vi "AddConfigureDialog.vi"(8 "Error In":errorcluster) -> (0 "Error Out":errorcluster)   [LabVIEW 2015]
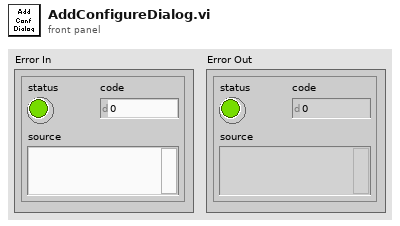
[diagram p1: front panel]
types:
  T1 = enum16{"Invalid Wire Rule", "Required", "Recommended", "Optional", "Dynamic Dispatch"}
  T2 = typedef "LVRectTypeDef.ctl" = cluster{"Left":i16, "Top":i16, "Right":i16, "Bottom":i16}
  T3 = enum16{"Invalid Wire Rule", "Required", "Recommended", "Optional", "Dynamic Dispatch"}[]
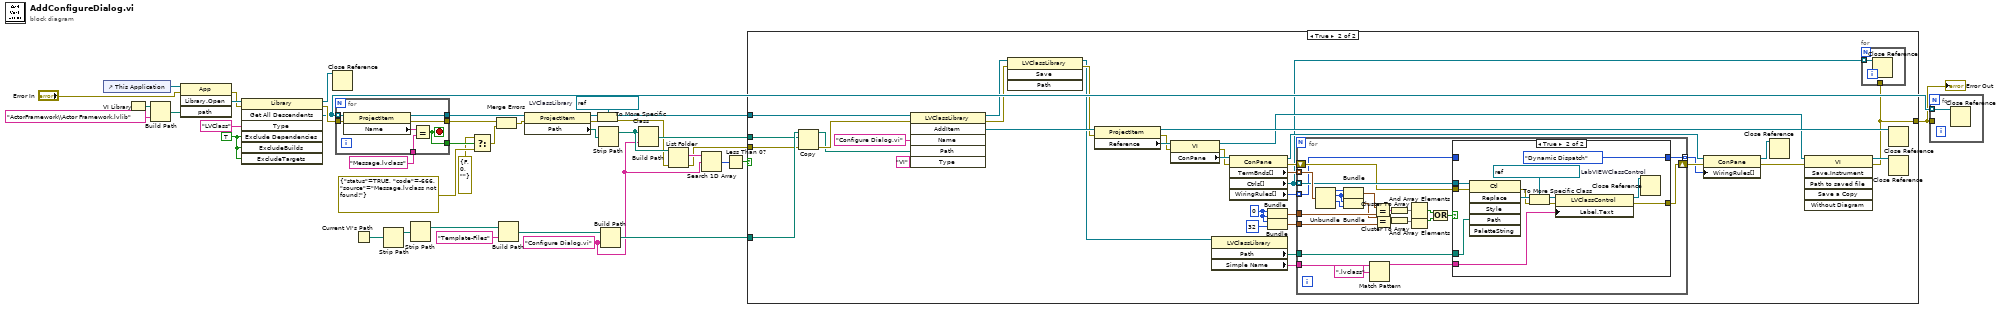
[diagram p0: block diagram]
diagram:
  w17 = refnum<vi> refnum  # LVClassLibrary
  w7 = "Configure Dialog.vi" ("name or relative path")
  w33 = TRUE ("ExcludeDependencies")
  n1 = control-ref of="This Application"() -> (w40:refnum<vi>)
  n2 = VI Library() -> (path=w39:path)
  n3 = Build Path(base path=w39, name or relative path="ActorFramework\\Actor Framework.lvlib") -> (appended path=w37:path)
  n4 = invoke class="App" method="Library.Open"(reference=w40, error in="Error In", "path"=w37) -> (error out=w34:errorcluster, "Open Library"=w35:refnum<vi>)  [unwired: 1 in, 2 out]
  n5 = invoke class="Library" method="Get All Descendents"(reference=w35, error in=w34, "Type"="LVClass", "Exclude Dependencies"=w33, "ExcludeBuilds"=w33, "ExcludeTargets"=w33) -> (reference out=w13:refnum<vi>, error out=w32:errorcluster, "All Descendents"=w12:refnum<vi>[])  [unwired: 1 in, 4 out]
  n6 = Close Reference(reference=w13) -> ()  [unwired: 1 in, 1 out]
  n7 = for {
    tunnel: w12 -> [w47] mode=indexing
    tunnel: "Message.lvclass" ("name") -> [w45]
    tunnel: [w44] -> w21
    tunnel: w32 -> [w43]
    tunnel: [w42] -> w26
    tunnel: [w41] -> w30
    stop <- w41 stop-if-true
    n8 = property class="ProjectItem"(reference=w47, error in=w43) -> (reference out=w44:refnum<vi>, error out=w42:errorcluster, "Name"=w46:string)
    n9 = Equal?(x=w46, y=w45) -> (x = y?=w41:bool)
  }
  n10 = Current VI's Path() -> (path=w25:path)
  n11 = Strip Path(path=w25) -> (stripped path=w24:path)  [unwired: 1 out]
  n12 = Strip Path(path=w24) -> (stripped path=w1:path)  [unwired: 1 out]
  n13 = Select(t=errorcluster {"status"=FALSE, "code"=0, "source"=""} ("error constant"), s=w30, f=errorcluster {"status"=TRUE, "code"=-666, "source"="Message.lvclass not found!"} ("error constant")) -> (s? t:f=w27:errorcluster)
  n14 = Merge Errors(w26, w27) -> (w20:errorcluster)
  n15 = Build Path(base path=w1, name or relative path="Template-Files") -> (appended path=w22:path)
  n16 = property class="ProjectItem"(reference=w21, error in=w20) -> (reference out=w16:refnum<vi>, error out=w14:errorcluster, "Path"=w18:path)
  n17 = To More Specific Class(target class=w17, reference=w16, error in=w14) -> (specific class reference=w15:refnum<vi>, error out=w9:errorcluster)
  n18 = Strip Path(path=w18) -> (stripped path=w10:path)  [unwired: 1 out]
  n19 = Build Path(base path=w22, name or relative path=w7) -> (appended path=w19:path)
  n20 = Build Path(base path=w10, name or relative path=w7) -> (appended path=w11:path)
  n21 = List Folder(path=w10, error in=w9) -> (filenames=w8:string[], error out=w6:errorcluster)  [unwired: 2 in, 2 out]
  n22 = Search 1D Array(1D array=w8, element=w7) -> (index of element=w5:i32)  [unwired: 1 in]
  n23 = Less Than 0?(x=w5) -> (x < 0?=w4:bool)
  n24 = case shown="True" w4 {
    tunnel: w19 -> [_ w78]
    tunnel: w15 -> [_ w76]
    tunnel: [w48 w51] -> w2
    tunnel: w11 -> [_ w50]
    tunnel: w6 -> [w48 w49]
    frame False {
    }
    frame True {
      w64 = i16 0
      n25 = Copy(8:w49, 10:w50, 11:w78) -> (0:w79:errorcluster, 3:w77:path)  [unwired: 2 in, 1 out]
      n26 = invoke class="LVClassLibrary" method="AddItem"(reference=w76, error in=w79, "Name"="Configure Dialog.vi", "Path"=w77, "Type"="VI") -> (reference out=w75:refnum<vi>, error out=w74:errorcluster, "AddItem"=w82:refnum<vi>)  [unwired: 1 in, 3 out]
      n27 = invoke class="LVClassLibrary" method="Save"(reference=w75, error in=w74) -> (reference out=w56:refnum<vi>, error out=w73:errorcluster)  [unwired: 2 in, 2 out]
      n28 = property class="ProjectItem"(reference=w82, error in=w73) -> (reference out=w81:refnum<vi>, error out=w57:errorcluster, "Reference"=w58:refnum<vi>)
      n29 = property class="VI"(reference=w58, error in=w57) -> (reference out=w55:refnum<vi>, error out=w71:errorcluster, "ConPane"=w72:refnum<vi>)
      n30 = property class="LVClassLibrary"(reference=w56) -> ("Path"=w65:path, "Simple Name"=w59:string)  [unwired: 1 in, 2 out]
      n31 = property class="ConPane"(reference=w72, error in=w71) -> (reference out=w61:refnum<vi>, error out=w69:errorcluster, "TermBnds[]"=w70:T2[], "Ctrls[]"=w52:refnum<vi>[], "WiringRules[]"=w63:T3)
      n32 = Bundle(w64, w64) -> (w67:cluster{i16, i16})  [unwired: 1 in]
      n33 = Bundle(w64, i16 32) -> (w66:cluster{i16, i16})  [unwired: 1 in]
      n34 = for {
        tunnel: w70 -> [w108] mode=indexing
        tunnel: w52 -> [w98] mode=indexing
        shift-right: [w92] -> w62
        shift-left: w69 -> [w97]
        tunnel: w67 -> [w105]
        tunnel: w66 -> [w103]
        tunnel: w65 -> [w93]
        tunnel: w63 -> [w89] mode=indexing
        tunnel: [w88] -> w60 mode=indexing
        tunnel: w59 -> [w87]
        n35 = Unbundle(w108) -> ("Left"=w107:i16, "Top"=w90:i16, "Right"=w91:i16)  [unwired: 1 out]
        n36 = Bundle("Left"=w107, "Top"=w90) -> (w106:cluster{"Left":i16, "Top":i16})  [unwired: 1 in]
        n37 = Bundle("Top"=w90, "Right"=w91) -> (w104:cluster{"Top":i16, "Right":i16})  [unwired: 1 in]
        n38 = Match Pattern(string=w87, regular expression=".lvclass") -> (before substring=w86:string)  [unwired: 1 in, 3 out]
        n39 = Equal?(x=w106, y=w105) -> (x = y?=w102:cluster{bool, bool})
        n40 = Equal?(x=w104, y=w103) -> (x = y?=w101:cluster{bool, bool})
        n41 = Cluster To Array(cluster=w102) -> (array=w100:bool[])
        n42 = Cluster To Array(cluster=w101) -> (array=w99:bool[])
        n43 = And Array Elements(Boolean array=w100) -> (logical AND=w96:bool)
        n44 = And Array Elements(Boolean array=w99) -> (logical AND=w95:bool)
        n45 = Or(x=w96, y=w95) -> (x .or. y?=w94:bool)
        n46 = case shown="True" w94 {
          tunnel: w98 -> [_ w122]
          tunnel: w97 -> [w110 w121]
          tunnel: [w110 w113] -> w92
          tunnel: w93 -> [_ w120]
          tunnel: w89 -> [w109 _]
          tunnel: [w109 T1."Dynamic Dispatch" ("Wire Rule")] -> w88
          tunnel: w86 -> [_ w111]
          frame False {
          }
          frame True {
            w118 = refnum<vi> refnum  # LabVIEWClassControl
            n47 = invoke class="Ctl" method="Replace"(reference=w122, error in=w121, "Path"=w120) -> (error out=w114:errorcluster, "Replace"=w117:refnum<vi>)  [unwired: 3 in, 4 out]
            n48 = To More Specific Class(target class=w118, reference=w117, error in=w114) -> (specific class reference=w116:refnum<vi>, error out=w115:errorcluster)
            n49 = property class="LVClassControl"(reference=w116, error in=w115, "Label.Text"=w111) -> (reference out=w112:refnum<vi>, error out=w113:errorcluster)
            n50 = Close Reference(reference=w112) -> ()  [unwired: 1 in, 1 out]
          }
        }
      }
      n51 = property class="ConPane"(reference=w61, error in=w62, "WiringRules[]"=w60) -> (reference out=w53:refnum<vi>, error out=w54:errorcluster)
      n52 = Close Reference(reference=w53) -> ()  [unwired: 1 in, 1 out]
      n53 = invoke class="VI" method="Save.Instrument"(reference=w55, error in=w54) -> (reference out=w80:refnum<vi>, error out=w51:errorcluster)  [unwired: 4 in, 4 out]
      n54 = for {
        tunnel: w52 -> [w123] mode=indexing
        tunnel: w51 -> [_]
        n55 = Close Reference(reference=w123) -> ()  [unwired: 1 in, 1 out]
      }
      n56 = Close Reference(reference=w81) -> ()  [unwired: 1 in, 1 out]
      n57 = Close Reference(reference=w80) -> ()  [unwired: 1 in, 1 out]
    }
  }
  "Error Out" <- w2
  n58 = for {
    tunnel: w2 -> [_]
    tunnel: w12 -> [w124] mode=indexing
    n59 = Close Reference(reference=w124) -> ()  [unwired: 1 in, 1 out]
  }
